vi "Mask Write Register.vi"(6 "timeout ms (1000)":i32=1000, 8 "error in (no error)":errorcluster, 9 "Masks":cluster{"And Mask":u8, "Or Mask":u8}, 10 "Address":u16, 11 "TCP Network Connection in":refnum<k5>) -> (0 "error out":errorcluster, 3 "TCP Network Connection out":refnum<k5>)   [LabVIEW 2023, in "Modbus TCP Micro.lvlib"]
uses:
  Modbus TCP Micro.lvlib
  Modbus Functions.ctl
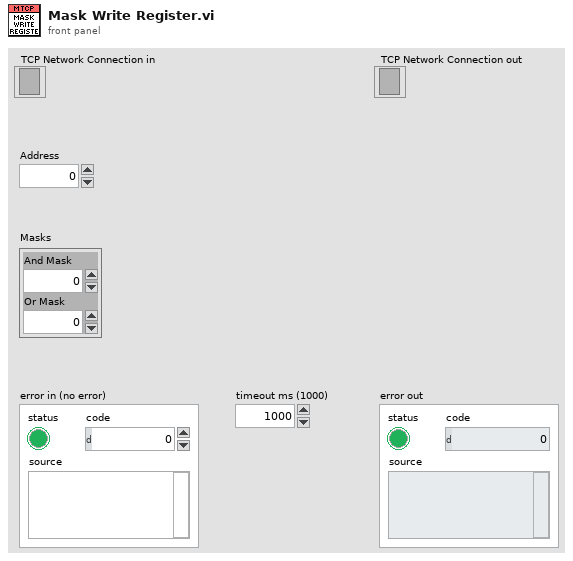
[diagram p1: front panel]
types:
  T1 = typedef "Modbus TCP Micro.lvlib/Modbus Functions.ctl" = u8
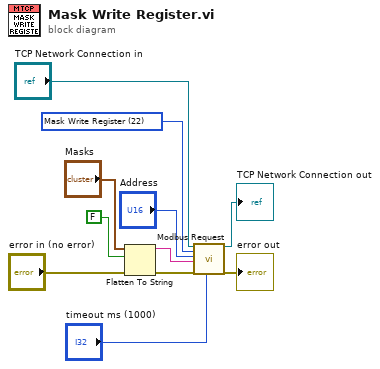
[diagram p0: block diagram]
diagram:
  w9 = T1 22 items=["None"=0, "Read Coil Status"=1, "Read Input Status"=2, "Read Holding Registers"=3, "Read Input Registers"=4, "Force Single Coil"=5, "Preset Single Register"=6, "Force Multiple Coils"=15, "Preset Multiple Registers"=16, "Mask Write Register"=22] ("Function Codes")
  n1 = Flatten To String(anything="Masks", prepend array or string size? (T)=FALSE, error in (no error)="error in (no error)") -> (data string=w4:string, error out=w5:errorcluster)  [unwired: 1 in, 1 out]
  n2 = call "Modbus Request.vi"("TCP Network Connection in"="TCP Network Connection in", "Function Codes"=w9, "Start Address"="Address", "Payload"=w4, "error in (no error)"=w5, "timeout ms (1000)"="timeout ms (1000)") -> ("TCP Network Connection out"=→"TCP Network Connection out":refnum<k5>, "error out"=→"error out":errorcluster)  [unwired: 8 in, 4 out]
